vi "GetSamplePictureName.vi"(8 "Error In":errorcluster, 10 "Array":i64[](array[numeric]), 11 "SampleName":string) -> (0 "Error Out":errorcluster, 3 "filename":string)   [LabVIEW 2019]
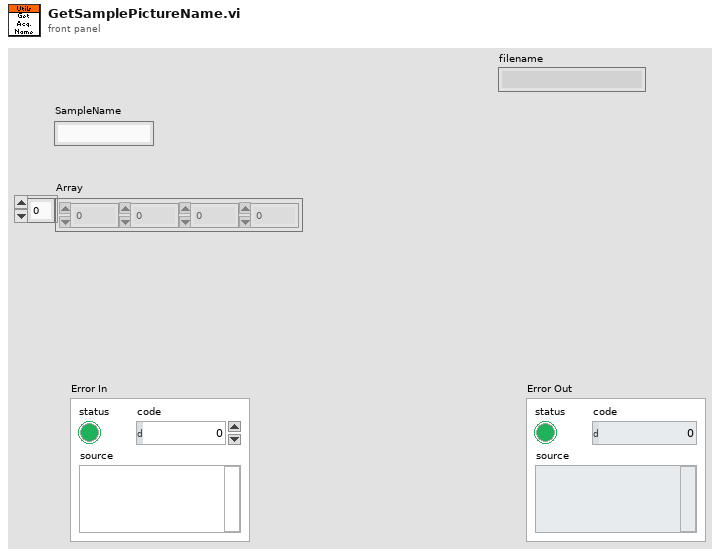
[diagram p1: front panel]
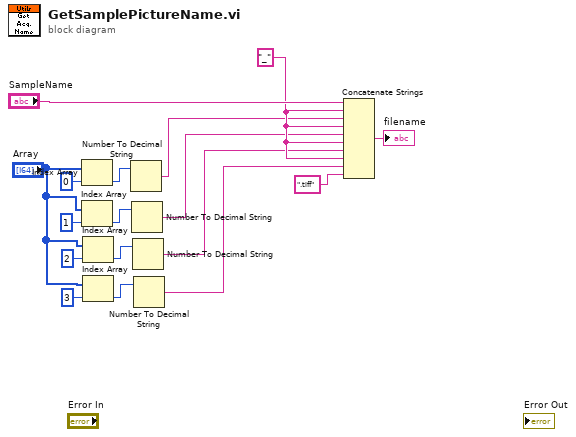
[diagram p0: block diagram]
diagram:
  w16 = "_"
  n1 = Index Array(array="Array", index=0) -> (element=w10:i64)
  n2 = Index Array(array="Array", index=1) -> (element=w8:i64)
  n3 = Index Array(array="Array", index=2) -> (element=w7:i64)
  n4 = Index Array(array="Array", index=3) -> (element=w6:i64)
  n5 = Number To Decimal String(number=w10) -> (decimal integer string=w9:string)  [unwired: 1 in]
  n6 = Number To Decimal String(number=w8) -> (decimal integer string=w5:string)  [unwired: 1 in]
  n7 = Number To Decimal String(number=w7) -> (decimal integer string=w4:string)  [unwired: 1 in]
  n8 = Number To Decimal String(number=w6) -> (decimal integer string=w3:string)  [unwired: 1 in]
  n9 = Concatenate Strings("SampleName", w16, w9, w16, w5, w16, w4, w16, w3, ".tiff") -> (→"filename":string)
